vi "XCP DAQ Read Single Point.vi"(8 "error in (no error)":errorcluster, 10 "Number of Sample":i32, 11 "DAQList in":refnum<class "DAQList.lvclass">) -> (0 "error out":errorcluster, 1 "Data":dbl[](array[numeric]), 3 "DAQList out":refnum<class "DAQList.lvclass">)   [LabVIEW 2019, in "XCP_DaqDtoId.lvlib" / "DAQList.lvclass"]
uses:
  DAQList.lvclass
  DAQList.lvclass/DAQList.ctl
  XnetRead/SubVI_MergeData2.vi
  XcpCommand/SendCommands.vi
  XcpCommand/FilterCommands.vi
  DatabaseGeneration/CreateCluster.vi
  DatabaseGeneration/CreateFrames.vi
  XnetRead/InitXnet.vi
  DatabaseGeneration/CreateSignals_SingleByte.vi
  DatabaseGeneration/SubVI_FilterDaqProcessorInfo.vi
  DatabaseGeneration/SubVI_FilterDaqResolutionInfo.vi
  XnetRead/InitMeaSplitInfo2.vi
  DatabaseGeneration/SubVI_SetMeasProp.vi
  DatabaseGeneration/SubVI_ProcessMaxOdtEntrySize.vi
  <vilib>/xnet/xnet.llb/XNET Create Session.vi
  <vilib>/xnet/xnet.llb/XNET Create Session (Frame Input Stream).vi
  <vilib>/xnet/xnet.llb/XNET Start.vi
  <vilib>/ECUMC/ECUMC.llb/MC DAQ List Initialize.vi
  <vilib>/ECUMC/ECUMC.llb/MC ECU Connect.vi
  <vilib>/ECUMC/ECUMC.llb/MC DAQ Start Stop.vi
  <vilib>/xnet/xnet.llb/XNET Read (Frame CAN).vi
  <vilib>/xnet/xnet.llb/XNET Clear.vi
  <vilib>/ECUMC/ECUMC.llb/MC Get Property.vi
  <vilib>/ECUMC/ECUMC.llb/MC Get Prop XCP CRO Id.vi
  <vilib>/ECUMC/ECUMC.llb/MC Get Prop XCP DTO Id.vi
  <vilib>/ECUMC/ECUMC.llb/MC Get Prop XCP CAN IO Mode.vi
  <vilib>/ECUMC/ECUMC.llb/MC Get Prop XCP Baud Rate 64.vi
  <vilib>/ECUMC/ECUMC.llb/MC Get Prop XCP FD Baud Rate 64.vi
  <vilib>/xnet/xnet.llb/XNET Database Create Object.vi
  <vilib>/xnet/xnet.llb/XNET Database Create (Cluster).vi
  <vilib>/Utility/error.llb/Error Cluster From Error Code.vi
  <vilib>/xnet/xnet.llb/XNET Database Create (Frame).vi
  <vilib>/Utility/file.llb/Application Directory.vi
  <vilib>/xnet/xnet.llb/XNET Database Save.vi
  DatabaseGeneration/CreateSignals.vi
  <vilib>/ECUMC/ECUMC.llb/MC Get Prop Meas Address.vi
  <vilib>/xnet/xnet.llb/XNET Database Create (Signal).vi
  <vilib>/xnet/xnet.llb/XNET Database Create (Subframe).vi
  <vilib>/ECUMC/ECUMC.llb/MC Get Prop Meas Data Type.vi
  <vilib>/xnet/xnet.llb/XNET Database Create (Dynamic Signal).vi
  <vilib>/ECUMC/ECUMC.llb/MC Get Prop Meas Comment.vi
  <vilib>/ECUMC/ECUMC.llb/MC Get Prop Meas Scaling Offset.vi
  <vilib>/ECUMC/ECUMC.llb/MC Get Prop Meas Scaling Factor.vi
  <vilib>/ECUMC/ECUMC.llb/MC Get Prop Meas Minimum.vi
  <vilib>/ECUMC/ECUMC.llb/MC Get Prop Meas Maximum.vi
  <vilib>/ECUMC/ECUMC.llb/MC Get Prop Meas Byte Order.vi
  <vilib>/ECUMC/ECUMC.llb/MC Get Prop Meas Unit.vi
  <vilib>/xnet/xnet.llb/XNET Create Session (Signal Input Waveform).vi
  TypeDef/Global.vi
  <vilib>/xnet/xnet.llb/XNET Read (Signal Waveform) .vi
panel:
  in  "timeout (1s)":dbl=1.0 format="%#_13g"
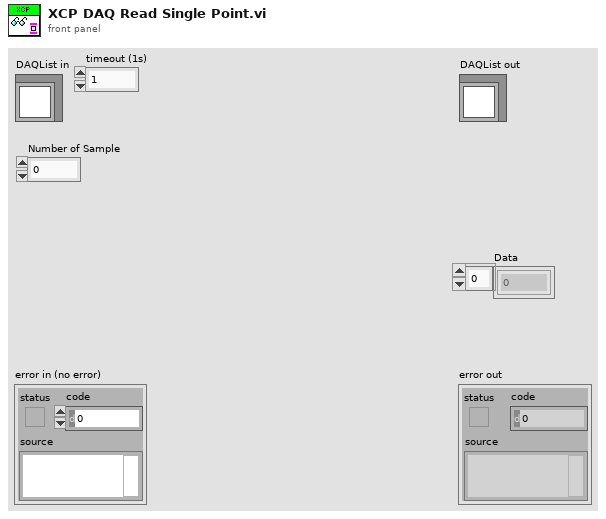
[diagram p1: front panel]
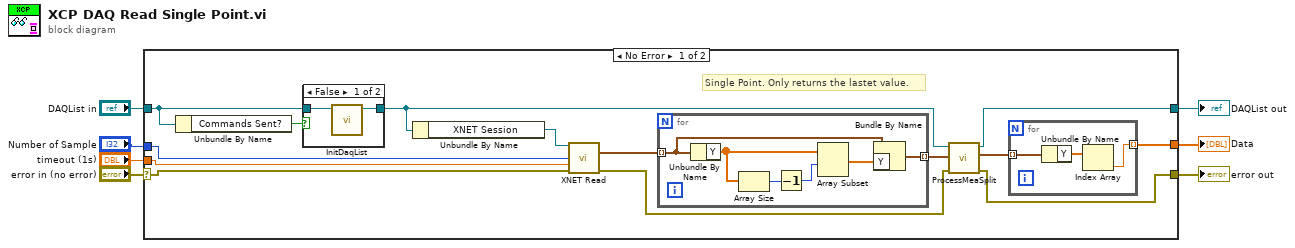
[diagram p0: block diagram]
diagram:
  n1 = case shown="No Error" "error in (no error)" {
    selector: "error in (no error)" -> [w19 w35]
    tunnel: [w13 w35] -> w6
    tunnel: [w18 w34] -> w4
    tunnel: "DAQList in" -> [w10 w34]
    tunnel: "Number of Sample" -> [w20 _]
    tunnel: [w12 _] -> w2
    tunnel: "timeout (1s)" -> [w8 _]
    frame No Error {
      # "Single Point. Only returns the lastet value."
      n2 = Unbundle By Name(w10) -> ("Commands Sent?"=w11:bool)
      n3 = case shown="False" w11 {
        tunnel: w10 -> [w23 w24]
        tunnel: [w22 w24] -> w9
        frame False {
          n4 = call "InitDaqList.vi"("DAQList in"=w23) -> ("DAQList out"=w22:refnum<class "DAQList.lvclass">)  [unwired: 9 in, 1 out]
        }
        frame True {
        }
      }
      n5 = Unbundle By Name(w9) -> ("XNET Session"=w21:refnum<k21>)
      n6 = call-poly <vilib>:"XNET Read.vi"("session in"=w21, "number to read (-1)"=w20, "timeout (0)"=w8, "error in (no error)"=w19) -> ("data"=w17:waveform(dbl)[], "error out"=w15:errorcluster)  [unwired: 10 out]
      n7 = for {
        tunnel: w17 -> [w33] mode=indexing
        tunnel: [w28] -> w16 mode=indexing
        n8 = Unbundle By Name(w33) -> ("Y"=w31:dbl[])
        n9 = Array Size(array=w31) -> (size(s)=w30:i32)
        n10 = Decrement(x=w30) -> (x-1=w29:i32)
        n11 = Array Subset(array=w31, index=w29) -> (w32:dbl[])  [unwired: 1 in]
        n12 = Bundle By Name(cluster=w33, "Y"=w32) -> (w28:waveform(dbl))
      }
      n13 = call "ProcessMeaSplit.vi"("error in (no error)"=w15, "Data In"=w16, "DAQList in"=w9) -> ("error out"=w13:errorcluster, "Data Out"=w14:waveform(dbl)[], "DAQList out"=w18:refnum<class "DAQList.lvclass">)  [unwired: 6 in]
      n14 = for {
        tunnel: w14 -> [w27] mode=indexing
        tunnel: [w25] -> w12 mode=indexing
        n15 = Unbundle By Name(w27) -> ("Y"=w26:dbl[])
        n16 = Index Array(array=w26) -> (element=w25:dbl)  [unwired: 1 in]
      }
    }
    frame Error {
    }
  }
  "error out" <- w6
  "DAQList out" <- w4
  "Data" <- w2
